vi "自动补全.vi"(8 "错误输入":errorcluster caption="错误输入（无错误）", 11 "引用":refnum<k24>) -> (0 "错误输出":errorcluster, 2 "引用输出 2":refnum<k24>, 3 "引用输出":refnum<k24>)   [LabVIEW 2018]
uses:
  ScintillaNET.dll
  AutocompleteMenu-ScintillaNET.dll
  System.Drawing
  System.Windows.Forms
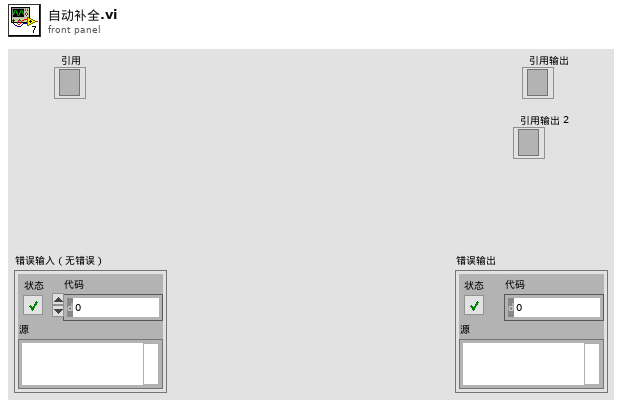
[diagram p1: front panel]
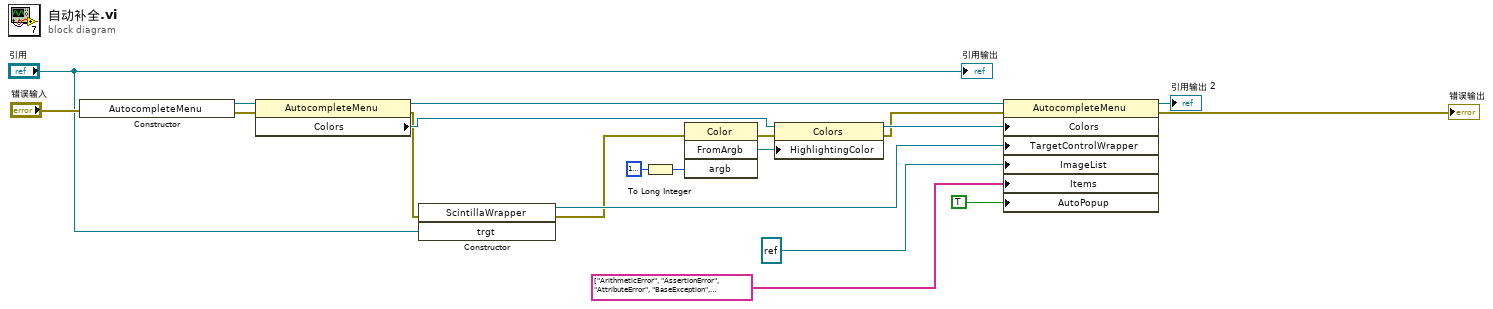
[diagram p0: block diagram]
diagram:
  n1 = constructor class="AutocompleteMenu"(error in="错误输入") -> (reference out=w6:refnum<k24>, error out=w14:errorcluster)  [unwired: 2 in, 1 out]
  n2 = property class="AutocompleteMenu"(reference=w6, error in=w14) -> (reference out=w5:refnum<k24>, error out=w9:errorcluster, "Colors"=w13:refnum<k24>)
  n3 = constructor class="ScintillaWrapper"(error in=w9, "trgt"="引用") -> (reference out=w11:refnum<k24>, error out=w10:errorcluster)  [unwired: 2 in, 2 out]
  n4 = To Long Integer(number=u32 16777216) -> (32bit integer=w19:i32)
  n5 = invoke class="Color" method="FromArgb"(error in=w10, "argb"=w19) -> (error out=w15:errorcluster, "FromArgb"=w17:refnum<k24>)  [unwired: 2 in, 2 out]
  n6 = property class="Colors"(reference=w13, error in=w15, "HighlightingColor"=w17) -> (reference out=w16:refnum<k24>, error out=w8:errorcluster)
  n7 = property class="AutocompleteMenu"(reference=w5, error in=w8, "Colors"=w16, "TargetControlWrapper"=w11, "ImageList"=refnum<k24> refnum, "Items"=string[] ["ArithmeticError", "AssertionError", "AttributeError", "BaseException", "BufferError", "BytesWarning", "DeprecationWarning", "EOFError", "EnvironmentError", "Exception", "False", "FloatingPointError", "FutureWarning", "GeneratorExit", "IOError", "ImportError", "ImportWarning", "IndentationError", "IndexError", "KeyError", "KeyboardInterrupt", "LookupError", "MemoryError", "NameError", "None", "NotImplementedError", "OSError", "OverflowError", "PendingDeprecationWarning", "ReferenceError", "RuntimeError", "RuntimeWarning", "StandardError", "StopIteration", "SyntaxError", "SyntaxWarning", "SystemError", "SystemExit", "TabError", "True", "TypeError", "UnboundLocalError", "UnicodeDecodeError", "UnicodeEncodeError", "UnicodeError", "UnicodeTranslateError", "UnicodeWarning", "UserWarning", "ValueError", "Warning", "ZeroDivisionError", "abs", "add", "all", "and", "any", "append", "apply", "as", "as_integer_ratio", "assert", "basestring", "bin", "bit_length", "bool", "break", "buffer", "bytearray", "bytes", "callable", "capitalize", "center", "chr", "class", "classmethod", "clear", "close", "cmp", "coerce", "compile", "complex", "conjugate", "continue", "copy", "count", "decode", "def", "del", "delattr", "deleter", "dict", "difference", "difference_update", "dir", "discard", "divmod", "elif", "else", "encode", "endswith", "enumerate", "eval", "except", "exec", "execfile", "expandtabs", "extend", "file", "fileno", "filter", "finally", "find", "float", "flush", "for", "format", "from", "fromhex", "fromkeys", "frozenset", "get", "getattr", "getter", "global", "globals", "has_key", "hasattr", "hash", "hex", "id", "if", "import", "in", "index", "indices", "input", "insert", "int", "intern", "intersection", "intersection_update", "is", "is_integer", "isalnum", "isalpha", "isatty", "isdecimal", "isdigit", "isdisjoint", "isinstance", "islower", "isnumeric", "isspace", "issubclass", "issubset", "issuperset", "istitle", "isupper", "items", "iter", "iteritems", "iterkeys", "itervalues", "join", "keys", "lambda", "len", "list", "ljust", "locals", "long", "lower", "lstrip", "map", "max", "memoryview", "min", "mro", "next", "not", "object", "oct", "open", "or", "ord", "partition", "pass", "pop", "popitem", "pow", "print", "property", "raise", "range", "raw_input", "read", "readinto", "readline", "readlines", "reduce", "reload", "remove", "replace", "repr", "return", "reverse", "reversed", "rfind", "rindex", "rjust", "round", "rpartition", "rsplit", "rstrip", "seek", "set", "setattr", "setdefault", "setter", "slice", "sort", "sorted", "split", "splitlines", "startswith", "staticmethod", "str", "strip", "sum", "super", "swapcase", "symmetric_difference", "symmetric_difference_update", "tell", "title", "tobytes", "tolist", "translate", "truncate", "try", "tuple", "type", "unichr", "unicode", "union", "update", "upper", "values", "vars", "viewitems", "viewkeys", "viewvalues", "while", "with", "write", "writelines", "xrange", "xreadlines", "yield", "zfill", "zip"] ("数组"), "AutoPopup"=TRUE) -> (reference out=→"引用输出 2":refnum<k24>, error out=→"错误输出":errorcluster)
  "引用输出" <- "引用"
